vi "File_permissions.vi"() -> ()   [LabVIEW 2010]
panel:
  out "permissions":i16
  in  "Permissions Bits set at creation":bool[](array[boolean])=[FALSE, TRUE, TRUE, FALSE, TRUE, TRUE, FALSE, FALSE, TRUE]
  out "Permissions Bits whilst file open":bool[](array[boolean])
  in  "deny mode (2)":T1(ring)=enum."deny none"
  out "Permissions Bits after closing file":bool[](array[boolean])
  # "others             group            user"
  # "x     w    r"
  # "x     w    r"
  # "x     w    r"
  # "others             group            user"
  # "x     w    r"
  # "x     w    r"
  # "x     w    r"
  # "Lock bit is 7 ^"
  # "others             group            user"
  # "x     w    r"
  # "x     w    r"
  # "x     w    r"
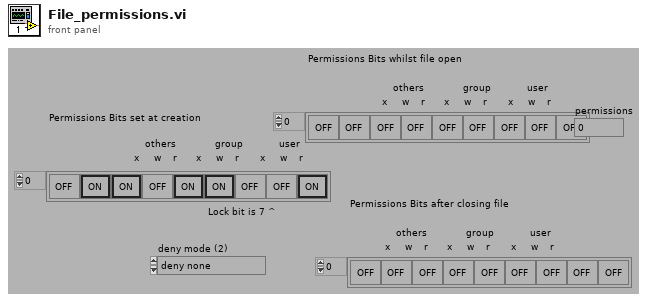
[diagram p1: front panel]
types:
  T1 = enum16{"deny read/write", "deny write-only", "deny none"}
  T2 = enum16{"open", "replace", "create", "open or create", "replace or create", "replace or create with confirmation"}
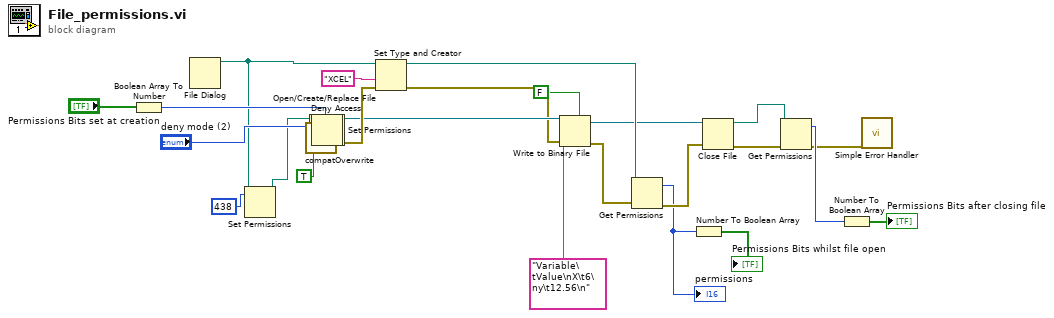
[diagram p0: block diagram]
diagram:
  n1 = Boolean Array To Number(Boolean array="Permissions Bits set at creation") -> (number=w11:u32)
  n2 = File Dialog() -> (3:w8:path)  [unwired: 7 in, 3 out]
  n3 = Set Permissions(7:i16 438 ("new permissions"), 11:w8) -> (3:w6:path)  [unwired: 3 in, 1 out]
  n4 = call <vilib>:"compatOverwrite.vi"("overwrite (F)"=TRUE) -> ("overwrite?"=w1:T2)
  n5 = Open/Create/Replace File(file path (use dialog)=w6, operation (0:open)=w1) -> (refnum out=w3:refnum<file>, error out=w2:errorcluster)  [unwired: 4 in, 1 out]
  n6 = Set Permissions(7:w11, 8:w2, 11:w6) -> (0:w4:errorcluster)  [unwired: 2 in, 1 out]
  n7 = Deny Access(4:w4, 6:"deny mode (2)", 7:w3) -> (0:w28:errorcluster, 3:w27:refnum<file>)
  n8 = Set Type and Creator(4:w28, 5:"XCEL" ("new creator"), 7:w8) -> (0:w9:errorcluster, 3:w17:path)  [unwired: 1 in]
  n9 = Write to Binary File(file (use dialog)=w27, data="Variable\tValue\nX\t6\ny\t12.56\n", error in=w9, 5:FALSE ("prepend array or string size? (T)")) -> (refnum out=w13:refnum<file>, error out=w18:errorcluster)  [unwired: 2 in, 1 out]
  n10 = Get Permissions(8:w18, 11:w17) -> (0:w16:errorcluster, 5:w15:i16)  [unwired: 3 out]
  "permissions" <- w15
  n11 = Number To Boolean Array(number=w15) -> (Boolean array=→"Permissions Bits whilst file open":bool[])
  n12 = Close File(refnum=w13, error in=w16) -> (path=w25:path, error out=w26:errorcluster)
  n13 = Get Permissions(8:w26, 11:w25) -> (0:w10:errorcluster, 5:w21:i16)  [unwired: 3 out]
  n14 = Number To Boolean Array(number=w21) -> (Boolean array=→"Permissions Bits after closing file":bool[])
  n15 = call <vilib>:"Simple Error Handler.vi"("error in (no error)"=w10) -> ()  [unwired: 4 in, 5 out]
